vi "testProcessEvent.vi"(8 "error in (no error)":errorcluster) -> (0 "error out":errorcluster)   [LabVIEW 2018]
doc: "Test the processEvent.vi."
uses:
  src/TcpServer/TcpServer.lvclass
  src/TcpServer/typedef/tcpPacketTypeDef.ctl
  <vilib>/addons/_JKI Toolkits/Caraya/classes/Assert/Assert Equal Value_Variant.vi
  <vilib>/addons/_JKI Toolkits/Caraya/classes/Test/Test.lvclass
  <vilib>/addons/_JKI Toolkits/Caraya/classes/Assert/Assert.lvclass
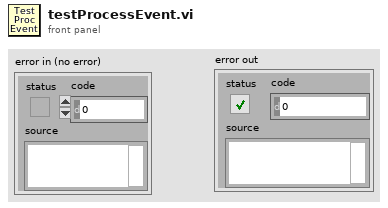
[diagram p1: front panel]
types:
  T1 = typedef "TcpServer.lvclass/tcpPacketTypeDef.ctl" = cluster{"packet":string, "firstPacket":bool, "firstConnection":bool}
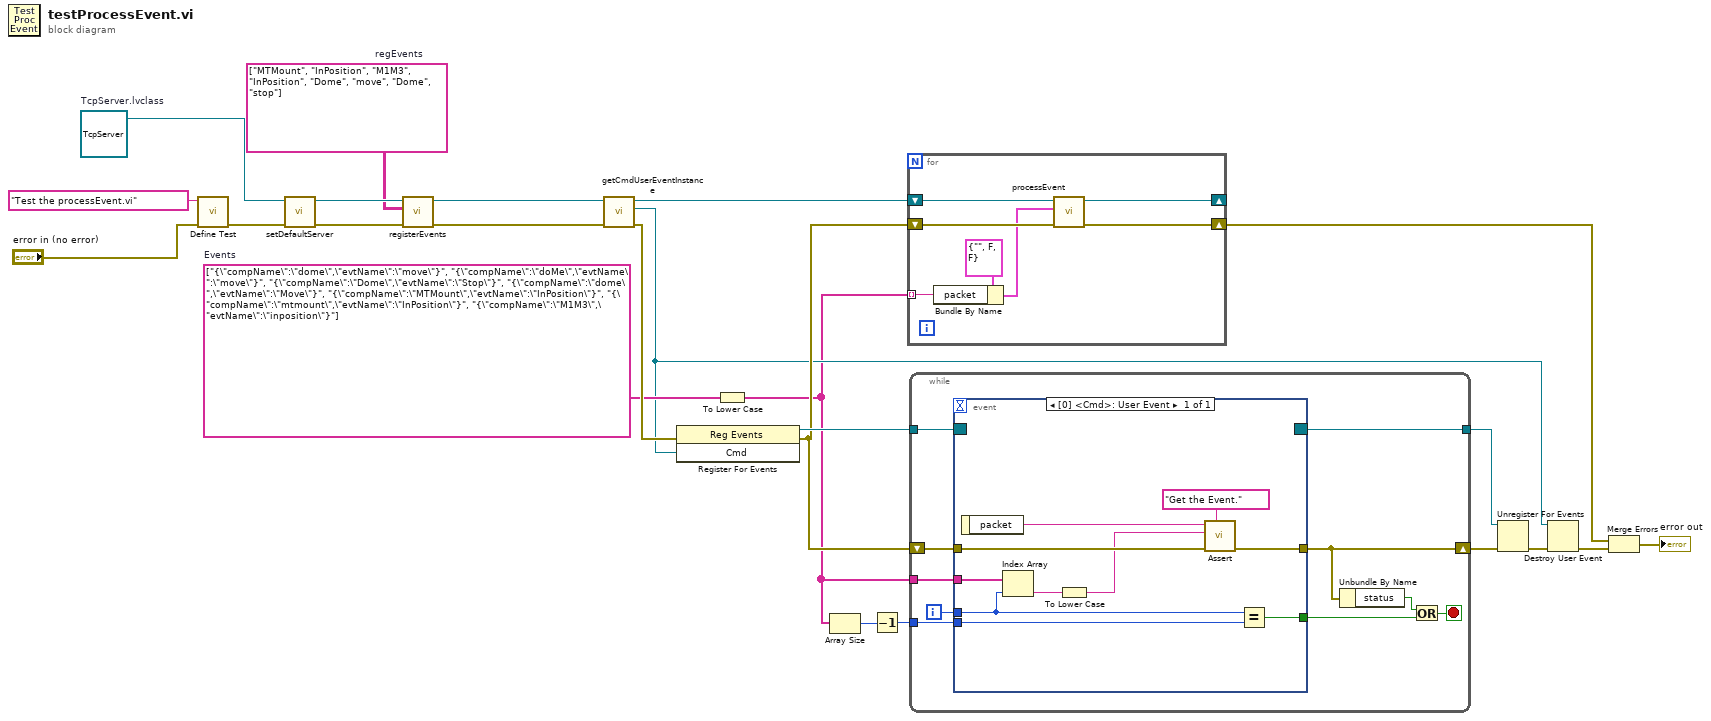
[diagram p0: block diagram]
diagram:
  w15 = string[][] [["MTMount", "InPosition"], ["M1M3", "InPosition"], ["Dome", "move"], ["Dome", "stop"]]  # regEvents
  w9 = string[] ["{\"compName\":\"dome\",\"evtName\":\"move\"}", "{\"compName\":\"doMe\",\"evtName\":\"move\"}", "{\"compName\":\"Dome\",\"evtName\":\"Stop\"}", "{\"compName\":\"dome\",\"evtName\":\"Move\"}", "{\"compName\":\"MTMount\",\"evtName\":\"InPosition\"}", "{\"compName\":\"mtmount\",\"evtName\":\"InPosition\"}", "{\"compName\":\"M1M3\",\"evtName\":\"inposition\"}"]  # Events
  w21 = refnum<class "TcpServer.lvclass"> refnum  # TcpServer.lvclass
  n1 = call <vilib>:"Define Test.vi"("error in (no error)"="error in (no error)", "Label (VI Title)"="Test the processEvent.vi") -> ("error out"=w23:errorcluster)  [unwired: 9 in]
  n2 = call "setDefaultServer.vi"("error in (no error)"=w23, "TcpServer.lvclass"=w21) -> ("error out"=w20:errorcluster, "tcpServer out"=w16:refnum<class "TcpServer.lvclass">)  [unwired: 8 in]
  n3 = call "registerEvents.vi"("error in (no error)"=w20, "registeredEvents"=w15, "tcpServer in"=w16) -> ("error out"=w17:errorcluster, "tcpServer out"=w13:refnum<class "TcpServer.lvclass">)  [unwired: 7 in]
  n4 = call "getCmdUserEventInstance.vi"("error in (no error)"=w17, "tcpServer in"=w13) -> ("error out"=w11:errorcluster, "Cmd"=w4:refnum<user-event>, "tcpServer out"=w12:refnum<class "TcpServer.lvclass">)  [unwired: 6 in, 1 out]
  n5 = register-events(error in=w11, w4) -> (reference out=w10:refnum<event-registration>, error out=w8:errorcluster)  [unwired: 1 in]
  n6 = To Lower Case(string=w9) -> (all lower case string=w1:string[])
  n7 = Array Size(array=w1) -> (size(s)=w14:i32)
  n8 = Decrement(x=w14) -> (x-1=w2:i32)
  n9 = for {
    tunnel: w1 -> [w27] mode=indexing
    shift-right: [w25] -> _
    shift-left: w12 -> [w29]
    shift-right: [w26] -> w18
    shift-left: w8 -> [w31]
    n10 = Bundle By Name(cluster=T1 {"packet"="", "firstPacket"=FALSE, "firstConnection"=FALSE} ("packetConnID"), "packet"=w27) -> (w28:T1)
    n11 = call "processEvent.vi"("error in (no error)"=w31, "tcpPacket"=w28, "tcpServer in"=w29) -> ("error out"=w26:errorcluster, "tcpServer out"=w25:refnum<class "TcpServer.lvclass">)  [unwired: 7 in]
  }
  n12 = while {
    tunnel: w10 -> [w40]
    tunnel: w1 -> [w39]
    shift-right: [w35] -> w7
    shift-left: w8 -> [w38]
    tunnel: [w37] -> w6
    tunnel: w2 -> [w36]
    i -> [w41]
    stop <- w33 stop-if-true
    n13 = event shown="[0] <Cmd>: User Event" {
      selector: w40 -> [_]
      dyn-events: [_] -> w37
      timeout: _ -> [_]
      tunnel: w41 -> [w44]
      tunnel: [w51] -> w32
      tunnel: w39 -> [w48]
      tunnel: w38 -> [w47]
      tunnel: [w45] -> w35
      tunnel: w36 -> [w43]
      event User Event {
        n14 = event-data() -> ("packet"=w49:string)  [unwired: 1 in]
        n15 = Index Array(array=w48, index=w44) -> (element=w46:string)
        n16 = To Lower Case(string=w46) -> (all lower case string=w42:string)
        n17 = call-poly <vilib>:"Assert.vi"("Label"="Get the Event.", "error in (no error)"=w47, "Y"=w42, "X"=w49) -> ("error out"=w45:errorcluster)  [unwired: 7 in]
        n18 = Equal?(x=w44, y=w43) -> (x = y?=w51:bool)
      }
    }
    n19 = Unbundle By Name(w35) -> ("status"=w34:bool)
    n20 = Or(x=w34, y=w32) -> (x .or. y?=w33:bool)
  }
  n21 = Unregister For Events(event registration refnum=w6, error in=w7) -> (error out=w5:errorcluster)
  n22 = Destroy User Event(user event=w4, error in=w5) -> (error out=w3:errorcluster)
  n23 = Merge Errors(w18, w3) -> (→"error out":errorcluster)
